vi "StoreChannelParams.vi"(8 "error in (no error)":errorcluster, 11 "ClassIn":refnum<class "NISTFGenPluginsBase.lvclass">) -> (0 "error out":errorcluster, 3 "ClassOut":refnum<class "NISTFGenPluginsBase.lvclass">)   [LabVIEW 2014, in "FGenPlugins.lvlib" / "NISTFGenPluginsBase.lvclass"]
uses:
  NISTFGenPluginsBase.lvclass
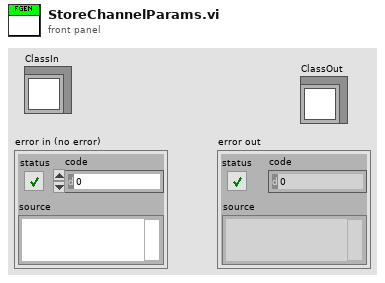
[diagram p1: front panel]
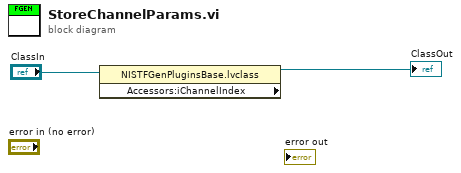
[diagram p0: block diagram]
diagram:
  n1 = property class="NISTFGenPluginsBase.lvclass" props=["Accessors:iChannelIndex"](reference="ClassIn") -> (reference out=→"ClassOut":refnum<class "NISTFGenPluginsBase.lvclass">)  [unwired: 1 in, 2 out]
